vi "CIE-Compute ASTF.vi"(0 "Mag":dbl[][](array[numeric]), 1 "Stimulus":dbl[](array[numeric]), 2 "Force no smoothing?":bool, 5 "Phase":dbl[][](array[numeric]), 7 "df (Hz)":dbl, 9 "Probe Mic Gain (dB)":dbl=50000.0, 11 "error in (no error)":errorcluster, 12 "Attenuation (dB)":dbl, 13 "Probe Tube Path":path) -> (3 "Smooth Params":T1={"Method"=enum."None", "MA"={"Iterations"=100, "Length"=3}, "Loess"={"Length"=21, "Type"=enum."Quadratic", "Robust"=TRUE}} {"Loess"."Length" min=1 step=1; "MA"."Length" min=1 step=1; "MA"."Iterations" min=1 step=1}, 4 "ASTF Mag":dbl[](array[numeric]), 6 "ASTF Phase":dbl[](array[numeric]), 8 "Frequency":dbl[](array[numeric]), 10 "Unsmoothed Mag":dbl[](array[numeric]), 15 "error out":errorcluster)   [LabVIEW 2020]
uses:
  Type Defs/Cal-Smoothing Parameters.ctl
  Utility VIs/Math VIs/LinSpace (x0-dx-npts).vi
  Utility VIs/Math VIs/FFT x(t) to dB,Degrees (1D).vi
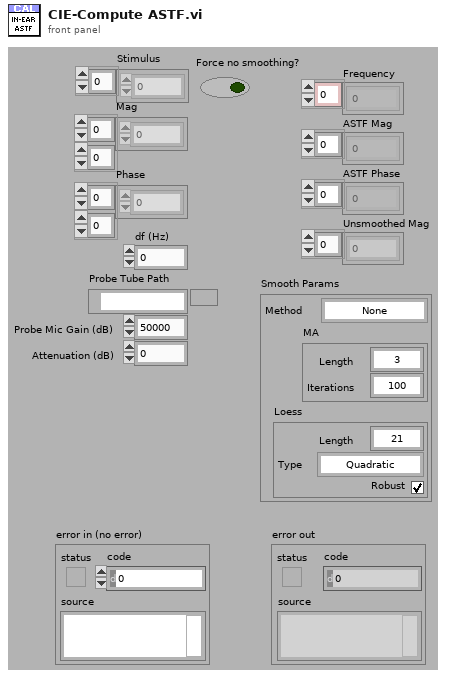
[diagram p1: front panel]
types:
  T1 = typedef "Cal-Smoothing Parameters.ctl" = cluster{"Method":enum16{"None", "Moving average", "Loess"}, "MA":cluster{"Iterations":i32, "Length":i32}, "Loess":cluster{"Length":i32, "Type":enum16{"Linear", "Quadratic"}, "Robust":bool}}
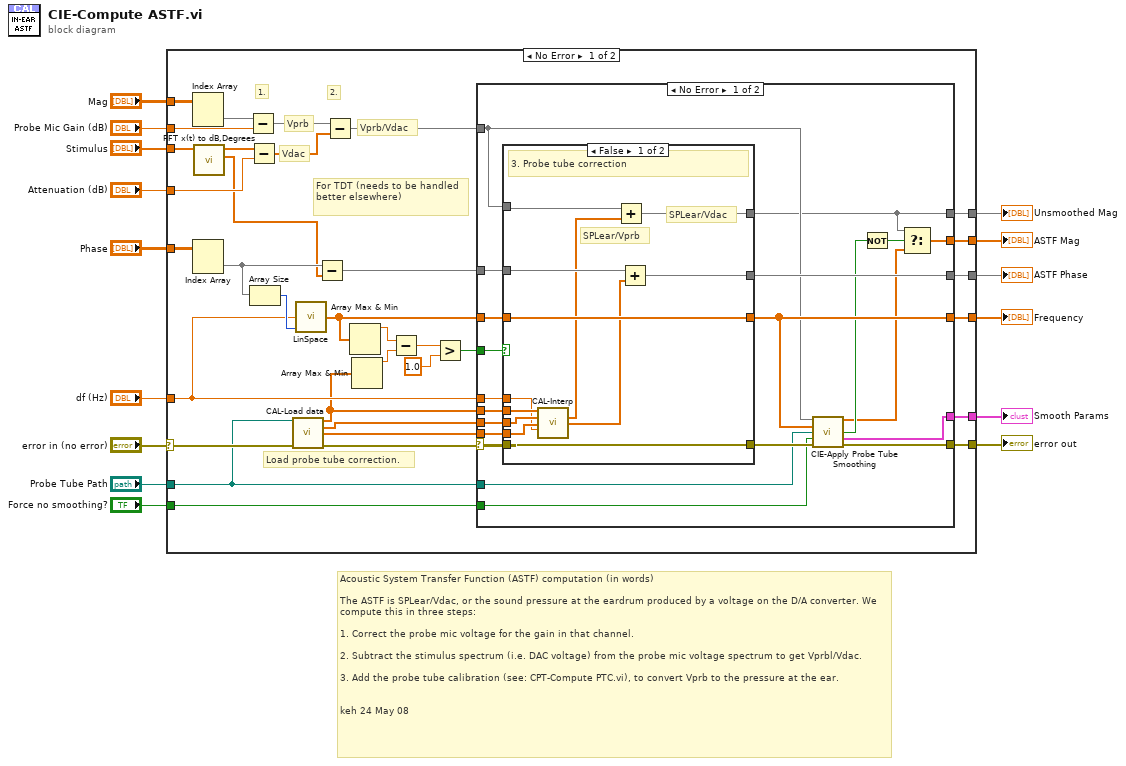
[diagram p0: block diagram]
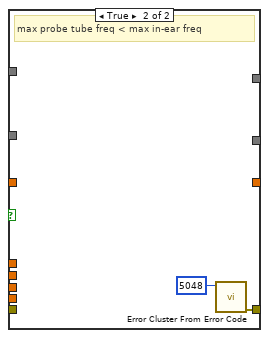
[diagram p2: hidden frame]
diagram:
  # "Acoustic System Transfer Function (ASTF) computation (in words)\n\nThe ASTF is SPLear/Vdac, or the sound pressure at the eardrum produced by a voltage on the D/A converter. We compute this in three steps:\n\n1. Correct the probe mic voltage for the gain in that channel.\n\n2. Subtract the stimulus spectrum (i.e. DAC voltage) from the probe mic voltage spectrum to get Vprbl/Vdac.\n\n3. Add the probe tube calibration (see: CPT-Compute PTC.vi), to convert Vprb to the pressure at the ear.\n\n\nkeh 24 May 08"
  n1 = case shown="No Error" "error in (no error)" {
    selector: "error in (no error)" -> [w45 w86]
    tunnel: "Mag" -> [w49 _]
    tunnel: "Phase" -> [w48 _]
    tunnel: [w44 _] -> w3
    tunnel: [w43 _] -> w13
    tunnel: "Stimulus" -> [w34 _]
    tunnel: "df (Hz)" -> [w26 _]
    tunnel: [w27 _] -> w9
    tunnel: "Probe Mic Gain (dB)" -> [w40 _]
    tunnel: [w38 w86] -> w7
    tunnel: "Attenuation (dB)" -> [w35 _]
    tunnel: "Probe Tube Path" -> [w20 _]
    tunnel: [w21 _] -> w4
    tunnel: "Force no smoothing?" -> [w19 _]
    tunnel: [w18 _] -> w1
    frame No Error {
      # "For TDT (needs to be handled better elsewhere)"
      # "Load probe tube correction."
      # "2."
      # "1."
      # "Vprb/Vdac"
      # "Vdac"
      # "Vprb"
      n2 = Index Array(array=w49) -> (element=w37:dbl[])  [unwired: 2 in]
      n3 = Index Array(array=w48) -> (element=w47:dbl[])  [unwired: 2 in]
      n4 = call-poly "FFT x(t) to dB,Degrees.vi"("X"=w34) -> ("+Freq Phase of FFT (degrees)"=w22:dbl[], "+Freq. Mag of FFT (dB rms)"=w32:dbl[])  [unwired: 8 in, 1 out]
      n5 = Subtract(x=w37, y=w40) -> (x-y=w41:dbl[])
      n6 = Subtract(x=w32, y=w35) -> (x-y=w33:dbl[])
      n7 = Array Size(array=w47) -> (size(s)=w46:i32)
      n8 = call "CAL-Load data.vi"("user path"=w20, "error in (no error)"=w45) -> ("Frequency (Hz)"=w25:dbl[], "Mag"=w24:dbl[], "Phase"=w23:dbl[], "error out"=w39:errorcluster)  [unwired: 6 in, 4 out]
      n9 = call-poly "LinSpace.vi"("npts"=w46, "dx"=w26) -> ("Array"=w28:dbl[])  [unwired: 2 in, 1 out]
      n10 = Subtract(x=w47, y=w22) -> (x-y=w42:dbl[])
      n11 = Subtract(x=w41, y=w33) -> (x-y=w36:dbl[])
      n12 = Array Max & Min(array=w28) -> (max value=w31:dbl)  [unwired: 3 out]
      n13 = Array Max & Min(array=w25) -> (max value=w30:dbl)  [unwired: 3 out]
      n14 = Subtract(x=w31, y=w30) -> (x-y=w29:dbl)
      n15 = Greater?(x=w29, y=1.0) -> (0:w17:bool)
      n16 = case shown="No Error" w39 {
        selector: w39 -> [w67 w85]
        tunnel: [w52 _] -> w44
        tunnel: [w70 _] -> w43
        tunnel: w42 -> [w69 _]
        tunnel: w17 -> [w68 _]
        tunnel: w36 -> [w59 _]
        tunnel: [w61 w85] -> w38
        tunnel: w28 -> [w66 _]
        tunnel: [w60 _] -> w27
        tunnel: w26 -> [w65 _]
        tunnel: w25 -> [w64 _]
        tunnel: w24 -> [w63 _]
        tunnel: w23 -> [w62 _]
        tunnel: [w56 _] -> w21
        tunnel: w20 -> [w57 _]
        tunnel: w19 -> [w51 _]
        tunnel: [w50 _] -> w18
        frame No Error {
          n17 = case shown="False" w68 {
            tunnel: w59 -> [w72 _]
            tunnel: [w82 _] -> w70
            tunnel: w69 -> [w81 _]
            tunnel: [w80 w84] -> w58
            tunnel: w67 -> [w80 _]
            tunnel: w66 -> [w79 _]
            tunnel: [w79 _] -> w60
            tunnel: w65 -> [w75 _]
            tunnel: w64 -> [w78 _]
            tunnel: w63 -> [w77 _]
            tunnel: w62 -> [w76 _]
            tunnel: [w71 _] -> w56
            frame False {
              # "SPLear/Vprb"
              # "SPLear/Vdac"
              # "3. Probe tube correction"
              n18 = call "CAL-Interp.vi"("Frequency (Hz)"=w78, "Magnitude (dB)"=w77, "Phase (degrees)"=w76, "df (Hz)"=w75) -> ("Interp Magnitude (dB)"=w74:dbl[], "Interp Phase (degrees)"=w73:dbl[])  [unwired: 8 in, 2 out]
              n19 = Add(x=w72, y=w74) -> (x+y=w71:dbl[])
              n20 = Add(x=w81, y=w73) -> (x+y=w82:dbl[])
            }
            frame True {
              # "max probe tube freq < max in-ear freq"
              n21 = call <vilib>:"Error Cluster From Error Code.vi"("error code (0)"=5048) -> ("error out"=w84:errorcluster)  [unwired: 8 in]
            }
          }
          n22 = call "CIE-Apply Probe Tube Smoothing.vi"("Vprb/Vdac"=w59, "Frequency (Hz)"=w60, "Probe Tube Path"=w57, "Override?"=w51, "error in (no error)"=w58) -> ("Smoothed Mag"=w53:dbl[], "Smoothed?"=w54:bool, "Smooth Params"=w50:T1, "error out"=w61:errorcluster)  [unwired: 7 in]
          n23 = Not(x=w54) -> (.not. x?=w55:bool)
          n24 = Select(t=w56, s=w55, f=w53) -> (s? t:f=w52:dbl[])
        }
        frame Error {
        }
      }
    }
    frame Error {
    }
  }
  "ASTF Mag" <- w3
  "ASTF Phase" <- w13
  "error out" <- w7
  "Frequency" <- w9
  "Unsmoothed Mag" <- w4
  "Smooth Params" <- w1
